vi "FABR-Init Analysis.vi"(0 "Params":T4={"Format"=20, "Stimulus"={"Destination"="", "Rep rate (/sec)"=0.0, "Alternate Polarity"=FALSE, "Duration (ms)"=0.0, "Ramp (ms)"=0.0, "Fs (Hz)"=0.0, "Frame size (s)"=0.0}, "Sequence"={"Freq"={"Expression"="", "Skip"=80}, "Level"={"Start (dB)"=20, "Stop (dB)"=80, "Step (dB)"=5}, "Order"=enum."Interleaved"}, "Response"={"Gain"=0.0, "Averages"=0, "Window (ms)"=0.0, "Fs (Hz)"=25000.0, "Save raw"=FALSE}, "Reject"=0.0} {"Sequence"."Level"."Start (dB)" step=5; "Response"."Window (ms)" format="%.2f"}, 5 "SCL in":cluster{T1[]}[](array[cluster]), 7 "Runtime in":T9, 11 "error in (no error)":errorcluster) -> (4 "Analysis":T2, 6 "SCL out":cluster{T1[]}[](array[cluster]), 8 "Runtime out":T9, 15 "error out":errorcluster)   [LabVIEW 2020]
uses:
  Typedefs/FABR-Runtime Data.ctl
  Typedefs/FABR-Stimulus Ticket.ctl
  Typedefs/FABR-Order.ctl
  Typedefs/FABR-Parameters.ctl
  Typedefs/FABR-Stimulus.ctl
  Typedefs/FABR-Sequence.ctl
  Typedefs/FABR-Response.ctl
  Typedefs/FABR-Analysis State.ctl
  Threshold Estimation VIs/ABR3-Threshold Estimation Result.ctl
  Typedefs/FABR-Stimulus Condition.ctl
  16d9c402-c510-48d4-9650-152cb1fd61c9.vi
panel:
  # "Freq X Level X Time"
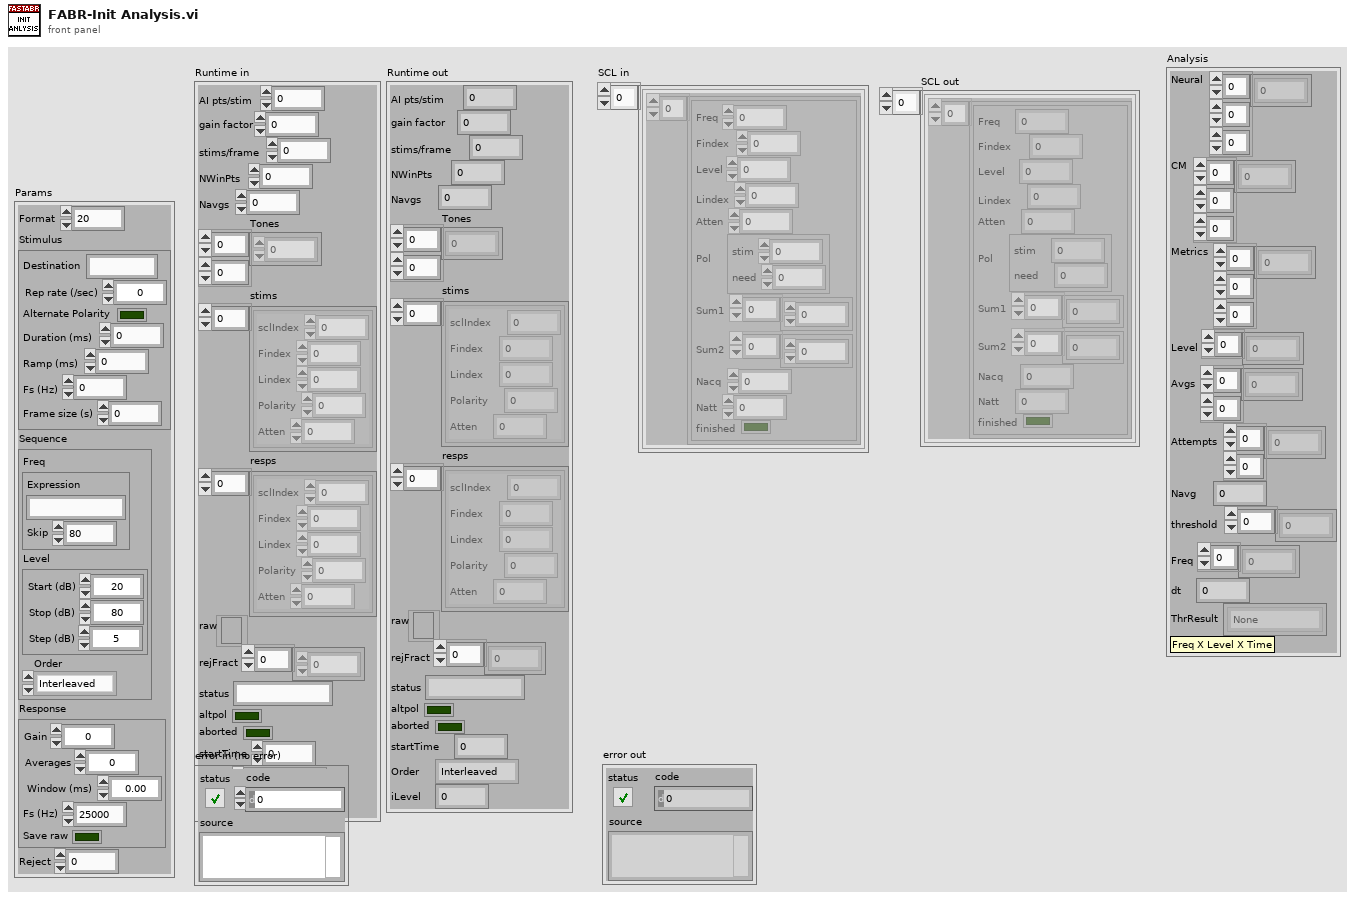
[diagram p1: front panel]
types:
  T1 = typedef "FABR-Stimulus Condition.ctl" = cluster{"Freq":dbl, "Findex":i32, "Level":dbl, "Lindex":i32, "Atten":dbl, "Pol":cluster{"stim":i32, "need":i32}, "Sum1":dbl[], "Sum2":dbl[], "Nacq":i32, "Natt":i32, "finished":bool}
  T2 = typedef "FABR-Analysis State.ctl" = cluster{"Neural":dbl[][][], "CM":dbl[][][], "Metrics":dbl[][][], "Level":dbl[], "Avgs":i32[][], "Attempts":i32[][], "Navg":i32, "threshold":dbl[], "Freq":dbl[], "dt":dbl, "ThrResult":T3[]}
  T3 = typedef "ABR3-Threshold Estimation Result.ctl" = enum16{"None", "Power", "Sigmoid", "Power (noisy)", "Suprathreshold", "Invalid"}
  T4 = typedef "FABR-Parameters.ctl" = cluster{"Format":i32, "Stimulus":T5, "Sequence":T6, "Response":T8, "Reject":dbl}
  T5 = typedef "FABR-Stimulus.ctl" = cluster{"Destination":string, "Rep rate (/sec)":dbl, "Alternate Polarity":bool, "Duration (ms)":dbl, "Ramp (ms)":dbl, "Fs (Hz)":dbl, "Frame size (s)":dbl}
  T6 = typedef "FABR-Sequence.ctl" = cluster{"Freq":cluster{"Expression":string, "Skip":i32}, "Level":cluster{"Start (dB)":i32, "Stop (dB)":i32, "Step (dB)":i32}, "Order":T7}
  T7 = typedef "FABR-Order.ctl" = enum16{"Interleaved", "Step level"}
  T8 = typedef "FABR-Response.ctl" = cluster{"Gain":dbl, "Averages":i32, "Window (ms)":sgl, "Fs (Hz)":dbl, "Save raw":bool}
  T9 = typedef "FABR-Runtime Data.ctl" = cluster{"AI pts/stim":i32, "gain factor":dbl, "stims/frame":i32, "NWinPts":i32, "Navgs":i32, "Tones":dbl[][], "stims":T10[], "resps":T10[], "raw":refnum<file>, "rejFract":dbl[], "status":string, "altpol":bool, "aborted":bool, "startTime":dbl, "Order":T7, "iLevel":i32}
  T10 = typedef "FABR-Stimulus Ticket.ctl" = cluster{"sclIndex":i32, "Findex":i32, "Lindex":i32, "Polarity":i32, "Atten":dbl}
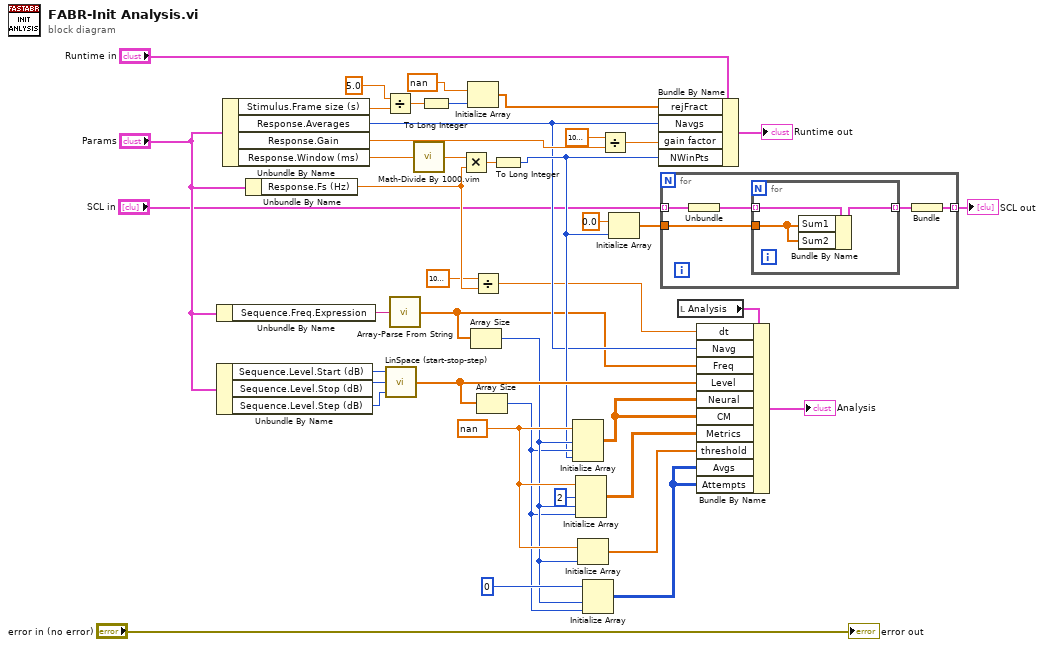
[diagram p0: block diagram]
diagram:
  w26 = nan ("element")
  n1 = Unbundle By Name("Params") -> ("Sequence.Freq.Expression"=w2:string)
  n2 = Unbundle By Name("Params") -> ("Sequence.Level.Start (dB)"=w40:i32, "Sequence.Level.Stop (dB)"=w41:i32, "Sequence.Level.Step (dB)"=w42:i32)
  n3 = Unbundle By Name("Params") -> ("Stimulus.Frame size (s)"=w8:dbl, "Response.Averages"=w14:i32, "Response.Gain"=w18:dbl, "Response.Window (ms)"=w38:sgl)
  n4 = Unbundle By Name("Params") -> ("Response.Fs (Hz)"=w13:dbl)
  n5 = Divide(x=5.0, y=w8) -> (x/y=w6:dbl)
  n6 = call "LinSpace (start-stop-step).vi"("Step"=w42, "Stop"=w41, "Start"=w40) -> ("Array"=w31:dbl[])  [unwired: 1 in, 1 out]
  n7 = call "Array-Parse From String.vi"("String"=w2) -> ("Array"=w1:dbl[])  [unwired: 13 in, 1 out]
  n8 = call "Math-Divide By 1000.vim"("X"=w38) -> ("1000X"=w39:dbl)
  n9 = To Long Integer(number=w6) -> (32bit integer=w5:i32)
  n10 = Multiply(x=w39, y=w13) -> (x*y=w37:dbl)
  n11 = Initialize Array(nan, w5) -> (w3:dbl[])
  n12 = Array Size(array=w1) -> (size(s)=w23:i32)
  n13 = Divide(x=1000000.0, y=w13) -> (x/y=w12:dbl)
  n14 = Array Size(array=w31) -> (size(s)=w22:i32)
  n15 = To Long Integer(number=w37) -> (32bit integer=w17:i32)
  n16 = Initialize Array(w26, w23, w22, w17) -> (w29:dbl[][][])
  n17 = Initialize Array(w26, 2 ("dimension size"), w23, w22) -> (w27:dbl[][][])
  n18 = Initialize Array(w26, w23) -> (w25:dbl[])
  n19 = Initialize Array(0, w23, w22) -> (w21:i32[][])
  n20 = Divide(x=1000000.0, y=w18) -> (x/y=w20:dbl)
  n21 = Initialize Array(0.0 ("element"), w17) -> (w15:dbl[])
  n22 = Bundle By Name(cluster="Runtime in", "rejFract"=w3, "Navgs"=w14, "gain factor"=w20, "NWinPts"=w17) -> (→"Runtime out":T9)
  n23 = for {
    tunnel: "SCL in" -> [w46] mode=indexing
    tunnel: w15 -> [w47]
    tunnel: [w43] -> w9 mode=indexing
    n24 = Unbundle(w46) -> (w45:T1[])
    n25 = for {
      tunnel: [w50] -> w44 mode=indexing
      tunnel: w47 -> [w49]
      tunnel: w45 -> [w48] mode=indexing
      n26 = Bundle By Name(cluster=w48, "Sum1"=w49, "Sum2"=w49) -> (w50:T1)
    }
    n27 = Bundle(w44) -> (w43:cluster{T1[]})  [unwired: 1 in]
  }
  "SCL out" <- w9
  n28 = local read "Analysis"() -> (w36:T2)
  n29 = Bundle By Name(cluster=w36, "dt"=w12, "Navg"=w14, "Freq"=w1, "Level"=w31, "Neural"=w29, "CM"=w29, "Metrics"=w27, "threshold"=w25, "Avgs"=w21, "Attempts"=w21) -> (→"Analysis":T2)
  "error out" <- "error in (no error)"
